vi "Spaltenindex finden.vi"(10 "Tabelle":string[][](array[string]), 11 "Regulärer Ausdruck":string) -> (3 "Tab spalte":i32)   [LabVIEW 2015, in "Sprachverwaltung.lvlib"]
uses:
  Sprachverwaltung.lvlib
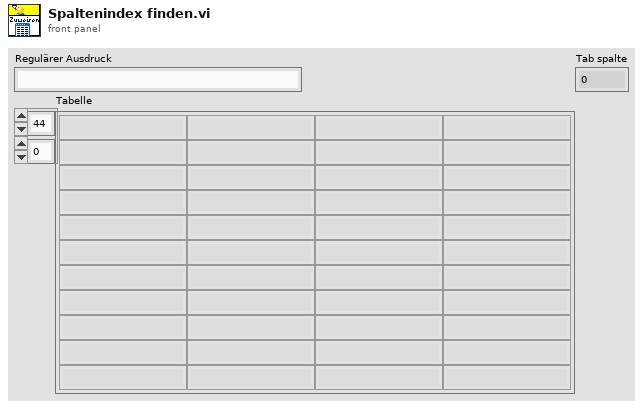
[diagram p1: front panel]
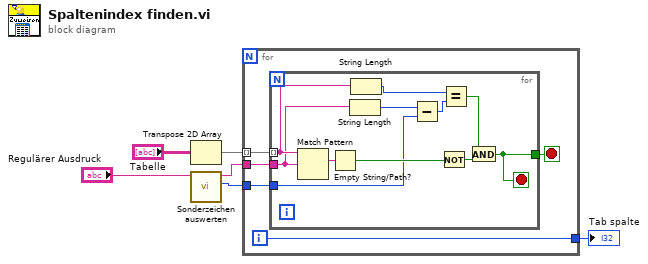
[diagram p0: block diagram]
diagram:
  n1 = Transpose 2D Array(2D array="Tabelle") -> (transposed array=w3:string[][])
  n2 = call "Sonderzeichen auswerten.vi"("String"="Regulärer Ausdruck") -> ("Anzahl"=w1:i32, "Suchstring"=w6:string)  [unwired: 9 in]
  n3 = for {
    tunnel: w6 -> [w11]
    tunnel: w3 -> [w10] mode=indexing
    tunnel: [w8] -> w4
    tunnel: w1 -> [w7]
    i -> [w8]
    stop <- w9 stop-if-true
    n4 = for {
      tunnel: w11 -> [w19]
      tunnel: w10 -> [w20] mode=indexing
      tunnel: [w14] -> w9
      tunnel: w7 -> [w12]
      stop <- w14 stop-if-true
      n5 = Match Pattern(string=w20, regular expression=w19) -> (match substring=w22:string)  [unwired: 1 in, 3 out]
      n6 = Empty String/Path?(string/path=w22) -> (empty?=w21:bool)
      n7 = String Length(string=w19) -> (length=w17:i32)
      n8 = String Length(string=w20) -> (length=w18:i32)
      n9 = Subtract(x=w17, y=w12) -> (x-y=w13:i32)
      n10 = Not(x=w21) -> (.not. x?=w16:bool)
      n11 = Equal?(x=w18, y=w13) -> (x = y?=w15:bool)
      n12 = And(x=w15, y=w16) -> (x .and. y?=w14:bool)
    }
  }
  "Tab spalte" <- w4
